vi "SetValueByItemName.vi"(0 "VI Reference In":refnum<vi>, 2 "delimiter (>>)":string=">>", 5 "Control Path":string, 7 "Item Name":string, 9 "Occurrence":i32=1, 11 "Error In":errorcluster) -> (4 "VI Reference Out":refnum<vi>, 15 "Error Out":errorcluster)   [LabVIEW 2016, in "Drona.lvlib" / "ControlValue.lvlib" / "StimulusMCListbox.lvlib"]
doc: "Sets value(signaling) for the multi column listbox control whose first column item name is specified with its occurrence. Set the value as 1 in occurrence to select the first occurrence of an item. \n\nThe input control name is given as a string , incase of path, use delimiters inbetween the path."
uses:
  StimulusMCListbox.lvlib
  <userlib>/_OpenG.lib/array/array.llb/Search 1D Array (String)__ogtk.vi
  <vilib>/Utility/error.llb/Error Cluster From Error Code.vi
  <vilib>/ErrorRing/Error Ring.xnode
  Drona.lvlib
  Get/GetControlRef/GetControlRef.lvlib
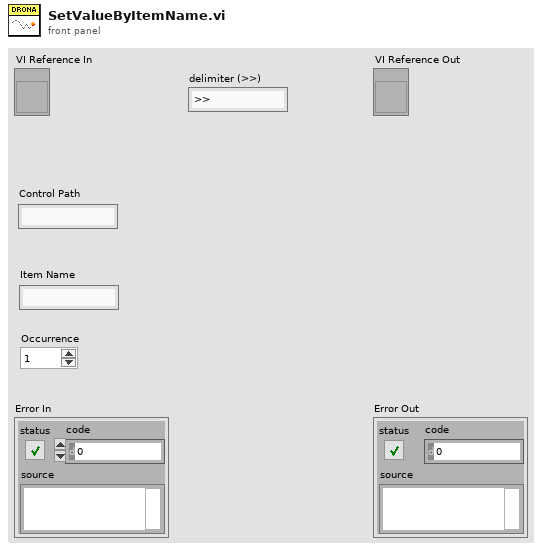
[diagram p1: front panel]
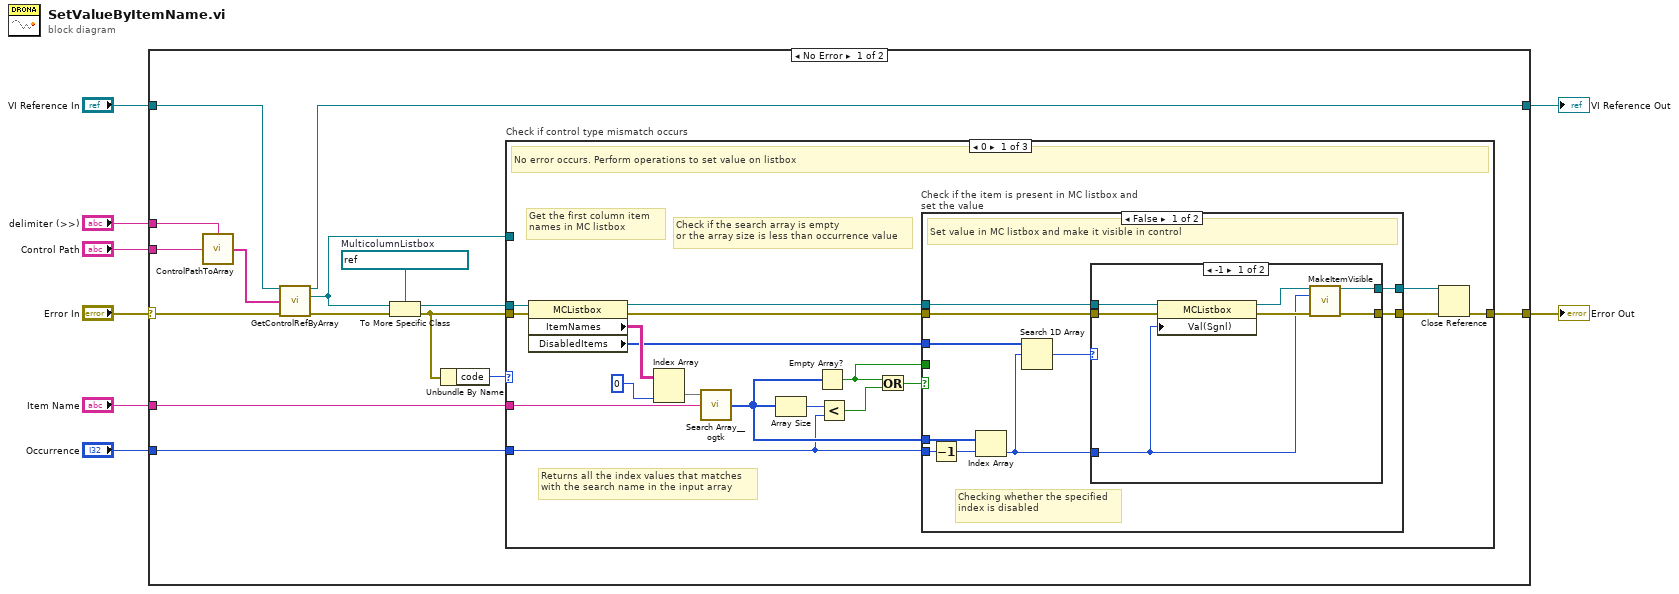
[diagram p0: block diagram]
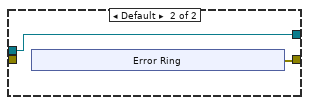
[diagram p2: hidden frame]
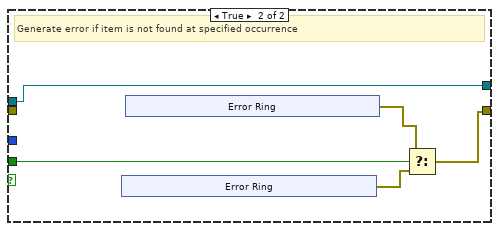
[diagram p3: hidden frame]
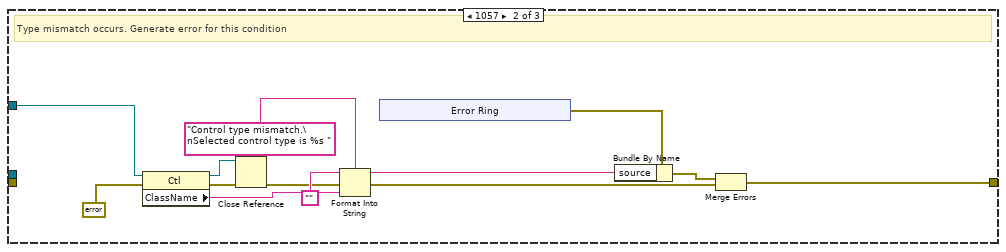
[diagram p4: hidden frame]
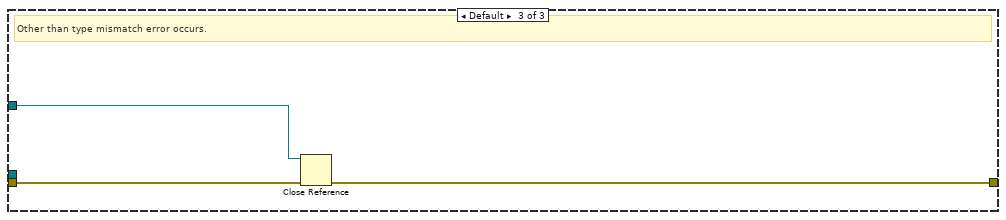
[diagram p5: hidden frame]
diagram:
  n1 = case shown="No Error" "Error In" {
    selector: "Error In" -> [w18 w103]
    tunnel: [w19 w103] -> w7
    tunnel: "VI Reference In" -> [w17 w102]
    tunnel: "Control Path" -> [w21 _]
    tunnel: [w14 w102] -> w4
    tunnel: "delimiter (>>)" -> [w20 _]
    tunnel: "Item Name" -> [w13 _]
    tunnel: "Occurrence" -> [w12 _]
    frame No Error {
      w23 = refnum<vi> refnum  # MulticolumnListbox
      n2 = call "ControlPathToArray.vi"("Control Name"=w21, "delimiter (>>)"=w20) -> ("Control Path"=w16:string[])
      n3 = call "GetControlRefByArray.vi"("VI Reference In"=w17, "Control Path"=w16, "error In"=w18) -> ("VI Reference Out"=w14:refnum<vi>, "Ctl Refnum"=w9:refnum<vi>, "error out"=w15:errorcluster)  [unwired: 10 in]
      n4 = To More Specific Class(target class=w23, reference=w9, error in=w15) -> (specific class reference=w22:refnum<vi>, error out=w11:errorcluster)
      n5 = Unbundle By Name(w11) -> ("code"=w10:i32)
      n6 = case "Check if control type mismatch occurs" shown="0" w10 {
        tunnel: w11 -> [w41 _ w101]
        tunnel: w22 -> [w40 _ _]
        tunnel: [w39 w81 w100] -> w19
        tunnel: w13 -> [w36 _ _]
        tunnel: w12 -> [w31 _ _]
        tunnel: w9 -> [_ w82 w99]
        frame 0 {
          # "Get the first column item \nnames in MC listbox"
          # "Check if the search array is empty \nor the array size is less than occurrence value"
          # "Returns all the index values that matches\nwith the search name in the input array"
          # "No error occurs. Perform operations to set value on listbox"
          n7 = property class="MCListbox"(reference=w40, error in=w41) -> (reference out=w29:refnum<vi>, error out=w30:errorcluster, "ItemNames"=w27:string[][], "DisabledItems"=w24:i32[])
          n8 = Index Array(array=w27, index (col)=0 ("disabled index (col)")) -> (element=w25:string[])  [unwired: 1 in]
          n9 = call-poly <userlib>:"Search Array__ogtk.vi"("Array"=w25, "Element Data"=w36) -> ("Indices of Elements"=w32:i32[])  [unwired: 7 in]
          n10 = Array Size(array=w32) -> (size(s)=w35:i32)
          n11 = Empty Array?(array=w32) -> (empty?=w28:bool)
          n12 = Less?(x=w35, y=w31) -> (x < y?=w34:bool)
          n13 = Or(x=w28, y=w34) -> (x .or. y?=w33:bool)
          n14 = case "Check if the item is present in MC listbox and set the value" shown="False" w33 {
            tunnel: [w51 w70] -> w38
            tunnel: [w50 w69] -> w37
            tunnel: w32 -> [w49 _]
            tunnel: w31 -> [w48 _]
            tunnel: w30 -> [w46 _]
            tunnel: w29 -> [w45 w69]
            tunnel: w28 -> [_ w68]
            tunnel: w24 -> [w44 _]
            frame False {
              # "Checking whether the specified index is disabled"
              # "Set value in MC listbox and make it visible in control"
              n15 = Decrement(x=w48) -> (x-1=w47:i32)
              n16 = Index Array(array=w49, index=w47) -> (element=w43:i32)
              n17 = Search 1D Array(1D array=w44, element=w43) -> (index of element=w42:i32)  [unwired: 1 in]
              n18 = case shown="-1" w42 {
                tunnel: [w57 w59] -> w51
                tunnel: [w56 w60] -> w50
                tunnel: w43 -> [w55 _]
                tunnel: w46 -> [w54 _]
                tunnel: w45 -> [w53 w60]
                frame -1 {
                  n19 = property class="MCListbox"(reference=w53, error in=w54, "Val(Sgnl)"=w55) -> (reference out=w52:refnum<vi>, error out=w58:errorcluster)
                  n20 = call "MakeItemVisible.vi"("MC ListBox Ref In"=w52, "Item Index"=w55, "Error In"=w58) -> ("MC ListBox Ref Out"=w56:refnum<vi>, "Error Out"=w57:errorcluster)  [unwired: 11 in]
                }
                frame Default {
                  n21 = xnode "Error Ring"() -> ("error out"=w59:errorcluster)
                }
              }
            }
            frame True {
              # "Generate error if item is not found at specified occurrence"
              n22 = xnode "Error Ring"() -> ("error out"=w66:errorcluster)
              n23 = xnode "Error Ring"() -> ("error out"=w67:errorcluster)
              n24 = Select(t=w67, s=w68, f=w66) -> (s? t:f=w70:errorcluster)
            }
          }
          n25 = Close Reference(reference=w37, error in (no error)=w38) -> (error out=w39:errorcluster)
        }
        frame 1057 {
          # "Type mismatch occurs. Generate error for this condition"
          n26 = property class="Ctl"(reference=w82, error in=errorcluster {"status"=FALSE, "code"=0, "source"=""} ("error out")) -> (reference out=w83:refnum<vi>, error out=w93:errorcluster, "ClassName"=w90:string)
          n27 = Close Reference(reference=w83, error in (no error)=w93) -> (error out=w84:errorcluster)
          n28 = Format Into String(format string="Control type mismatch.\nSelected control type is %s ", initial string="", error in=w84, w90) -> (resulting string=w87:string, error out=w85:errorcluster)
          n29 = xnode "Error Ring"() -> ("error out"=w88:errorcluster)
          n30 = Bundle By Name(cluster=w88, "source"=w87) -> (w86:errorcluster)
          n31 = Merge Errors(w86, w85) -> (w81:errorcluster)
        }
        frame Default {
          # "Other than type mismatch error occurs."
          n32 = Close Reference(reference=w99, error in (no error)=w101) -> (error out=w100:errorcluster)
        }
      }
    }
    frame Error {
    }
  }
  "Error Out" <- w7
  "VI Reference Out" <- w4
